vi "Load Actor.vi"   [LabVIEW 2020, in "RefNums and UICtrl.lvclass"]
uses:
  RefNums and UICtrl.lvclass
  <vilib>/MGI/Monitored Actor/Monitored Actor/Monitored Actor/Monitored Actor.lvclass
  C:/Program Files (x86)/National Instruments/LabVIEW 2020/vi.lib/ActorFramework/Actor/Actor.lvclass
  RefNums and UICtrl.lvclass/RefNums and UICtrl.ctl
  <vilib>/ActorFramework/Actor/Actor.lvclass
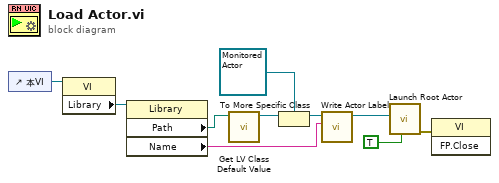
[diagram p0: block diagram]
diagram:
  n1 = control-ref of="本VI"() -> (w10:refnum<vi>)
  n2 = property class="VI"(reference=w10) -> ("Library"=w9:refnum<vi>)  [unwired: 1 in, 2 out]
  n3 = property class="Library"(reference=w9) -> ("Path"=w8:path, "Name"=w1:string)  [unwired: 1 in, 2 out]
  n4 = call <vilib>:"Get LV Class Default Value.vi"("class path"=w8) -> ("object"=w5:refnum<class>)  [unwired: 9 in, 1 out]
  n5 = To More Specific Class(target class=refnum<class "Monitored Actor.lvclass"> refnum ("Monitored Actor in"), reference=w5) -> (specific class reference=w3:refnum<class "Monitored Actor.lvclass">)  [unwired: 1 in, 1 out]
  n6 = call-dynamic "Write Actor Label.vi"("Actor Label"=w1, "Monitored Actor in"=w3) -> ("Monitored Actor out"=w6:refnum<class "Monitored Actor.lvclass">)  [unwired: 8 in, 1 out]
  n7 = call <vilib>:"Launch Root Actor.vi"("Open Actor Core front panel? (F)"=TRUE, "Actor"=w6) -> ("error out"=w7:errorcluster)  [unwired: 8 in, 1 out]
  n8 = invoke class="VI" method="FP.Close"(error in=w7) -> ()  [unwired: 2 in, 3 out]
